vi "Config editor for 19 cluster.vi"() -> ()   [LabVIEW 2022 SP3]
uses:
  085b3232-e767-4131-a9f9-8eb3103b6023.vi
  <vilib>/Utility/file.llb/Read Delimited Spreadsheet (string).vi
  <vilib>/Utility/file.llb/Write Delimited Spreadsheet (string).vi
panel:
  out "AI config 2":T1(array[cluster])=[{"Channel_Name"="G_PT_Press_1", "Channel_Number"="PXI2Slot5/ai1", "Pre_Scale_min"=0.0, "Pre_Scale_max"=10.0, "Sensor_min"=0.0, "Sensor_max"=100.0, "Units"="barg", "VI Category"="AI_V_1KHZ"}, {"Channel_Name"="G_PT_Press_2", "Channel_Number"="PXI2Slot4/ai6", "Pre_Scale_min"=0.004, "Pre_Scale_max"=0.02, "Sensor_min"=0.0, "Sensor_max"=100.0, "Units"="barg", "VI Category"="AI_C_NRT"}, {"Channel_Name"="I_PT(P)_1", "Channel_Number"="PXI2Slot2/ai0", "Pre_Scale_min"=0.004, "Pre_Scale_max"=0.02, "Sensor_min"=0.0, "Sensor_max"=100.0, "Units"="barg", "VI Category"="AI_C_RT"}, {"Channel_Name"="I_PT(P)_2", "Channel_Number"="PXI2Slot2/ai1", "Pre_Scale_min"=0.004, "Pre_Scale_max"=0.02, "Sensor_min"=0.0, "Sensor_max"=100.0, "Units"="barg", "VI Category"="AI_C_RT"}, {"Channel_Name"="I_PT(P)_3", "Channel_Number"="PXI2Slot2/ai2", "Pre_Scale_min"=0.004, "Pre_Scale_max"=0.02, "Sensor_min"=0.0, "Sensor_max"=100.0, "Units"="barg", "VI Category"="AI_C_RT"}, {"Channel_Name"="I_PT(P)_4", "Channel_Number"="PXI2Slot2/ai3", "Pre_Scale_min"=0.004, "Pre_Scale_max"=0.02, "Sensor_min"=0.0, "Sensor_max"=100.0, "Units"="barg", "VI Category"="AI_C_RT"}, {"Channel_Name"="I_PT(P)_5", "Channel_Number"="PXI2Slot2/ai4", "Pre_Scale_min"=0.004, "Pre_Scale_max"=0.02, "Sensor_min"=0.0, "Sensor_max"=100.0, "Units"="barg", "VI Category"="AI_C_RT"}, {"Channel_Name"="I_PT(P)_6", "Channel_Number"="PXI2Slot2/ai5", "Pre_Scale_min"=0.004, "Pre_Scale_max"=0.02, "Sensor_min"=0.0, "Sensor_max"=100.0, "Units"="barg", "VI Category"="AI_C_RT"}, {"Channel_Name"="I_PT(P)_7", "Channel_Number"="PXI2Slot2/ai6", "Pre_Scale_min"=0.004, "Pre_Scale_max"=0.02, "Sensor_min"=0.0, "Sensor_max"=100.0, "Units"="barg", "VI Category"="AI_C_RT"}, {"Channel_Name"="I_PT(P)_8", "Channel_Number"="PXI2Slot2/ai7", "Pre_Scale_min"=0.004, "Pre_Scale_max"=0.02, "Sensor_min"=0.0, "Sensor_max"=100.0, "Units"="barg", "VI Category"="AI_C_RT"}, {"Channel_Name"="I_PT(P)_9", "Channel_Number"="PXI2Slot2/ai8", "Pre_Scale_min"=0.004, "Pre_Scale_max"=0.02, "Sensor_min"=0.0, "Sensor_max"=100.0, "Units"="barg", "VI Category"="AI_C_RT"}, {"Channel_Name"="I_PT(P)_10", "Channel_Number"="PXI2Slot2/ai9", "Pre_Scale_min"=0.004, "Pre_Scale_max"=0.02, "Sensor_min"=0.0, "Sensor_max"=100.0, "Units"="barg", "VI Category"="AI_C_RT"}, {"Channel_Name"="I_PT(P)_11", "Channel_Number"="PXI2Slot2/ai10", "Pre_Scale_min"=0.004, "Pre_Scale_max"=0.02, "Sensor_min"=0.0, "Sensor_max"=100.0, "Units"="barg", "VI Category"="AI_C_RT"}, {"Channel_Name"="I_PT(P)_12", "Channel_Number"="PXI2Slot2/ai11", "Pre_Scale_min"=0.004, "Pre_Scale_max"=0.02, "Sensor_min"=0.0, "Sensor_max"=100.0, "Units"="barg", "VI Category"="AI_C_RT"}, {"Channel_Name"="I_PT(P)_13", "Channel_Number"="PXI2Slot2/ai12", "Pre_Scale_min"=0.004, "Pre_Scale_max"=0.02, "Sensor_min"=0.0, "Sensor_max"=100.0, "Units"="barg", "VI Category"="AI_C_RT"}, {"Channel_Name"="I_PT(P)_14", "Channel_Number"="PXI2Slot2/ai13", "Pre_Scale_min"=0.004, "Pre_Scale_max"=0.02, "Sensor_min"=0.0, "Sensor_max"=100.0, "Units"="barg", "VI Category"="AI_C_RT"}, {"Channel_Name"="I_PT(P)_15", "Channel_Number"="PXI2Slot2/ai14", "Pre_Scale_min"=0.004, "Pre_Scale_max"=0.02, "Sensor_min"=0.0, "Sensor_max"=100.0, "Units"="barg", "VI Category"="AI_C_RT"}, {"Channel_Name"="I_PT(P)_16", "Channel_Number"="PXI2Slot2/ai15", "Pre_Scale_min"=0.004, "Pre_Scale_max"=0.02, "Sensor_min"=0.0, "Sensor_max"=100.0, "Units"="barg", "VI Category"="AI_C_RT"}, {"Channel_Name"="I_PT(P)_17", "Channel_Number"="PXI2Slot2/ai16", "Pre_Scale_min"=0.004, "Pre_Scale_max"=0.02, "Sensor_min"=0.0, "Sensor_max"=100.0, "Units"="barg", "VI Category"="AI_C_RT"}, {"Channel_Name"="I_PT(P)_18", "Channel_Number"="PXI2Slot2/ai17", "Pre_Scale_min"=0.004, "Pre_Scale_max"=0.02, "Sensor_min"=0.0, "Sensor_max"=100.0, "Units"="barg", "VI Category"="AI_C_RT"}, {"Channel_Name"="I_PT(P)_19", "Channel_Number"="PXI2Slot2/ai18", "Pre_Scale_min"=0.004, "Pre_Scale_max"=0.02, "Sensor_min"=0.0, "Sensor_max"=100.0, "Units"="barg", "VI Category"="AI_C_RT"}, {"Channel_Name"="I_PT(Red)_1", "Channel_Number"="PXI2Slot2/ai19", "Pre_Scale_min"=0.004, "Pre_Scale_max"=0.02, "Sensor_min"=0.0, "Sensor_max"=100.0, "Units"="barg", "VI Category"="AI_C_RT"}, {"Channel_Name"="I_PT(Red)_2", "Channel_Number"="PXI2Slot2/ai20", "Pre_Scale_min"=0.004, "Pre_Scale_max"=0.02, "Sensor_min"=0.0, "Sensor_max"=100.0, "Units"="barg", "VI Category"="AI_C_RT"}, {"Channel_Name"="I_PT(Red)_3", "Channel_Number"="PXI2Slot2/ai21", "Pre_Scale_min"=0.004, "Pre_Scale_max"=0.02, "Sensor_min"=0.0, "Sensor_max"=100.0, "Units"="barg", "VI Category"="AI_C_RT"}, {"Channel_Name"="I_PT(Red)_4", "Channel_Number"="PXI2Slot2/ai22", "Pre_Scale_min"=0.004, "Pre_Scale_max"=0.02, "Sensor_min"=0.0, "Sensor_max"=100.0, "Units"="barg", "VI Category"="AI_C_RT"}, {"Channel_Name"="I_PT(Red)_5", "Channel_Number"="PXI2Slot2/ai23", "Pre_Scale_min"=0.004, "Pre_Scale_max"=0.02, "Sensor_min"=0.0, "Sensor_max"=100.0, "Units"="barg", "VI Category"="AI_C_RT"}, {"Channel_Name"="I_PT(Red)_6", "Channel_Number"="PXI2Slot2/ai24", "Pre_Scale_min"=0.004, "Pre_Scale_max"=0.02, "Sensor_min"=0.0, "Sensor_max"=100.0, "Units"="barg", "VI Category"="AI_C_RT"}, {"Channel_Name"="I_PT(Red)_7", "Channel_Number"="PXI2Slot2/ai25", "Pre_Scale_min"=0.004, "Pre_Scale_max"=0.02, "Sensor_min"=0.0, "Sensor_max"=100.0, "Units"="barg", "VI Category"="AI_C_RT"}, {"Channel_Name"="I_PT(Red)_8", "Channel_Number"="PXI2Slot2/ai26", "Pre_Scale_min"=0.004, "Pre_Scale_max"=0.02, "Sensor_min"=0.0, "Sensor_max"=100.0, "Units"="barg", "VI Category"="AI_C_RT"}, {"Channel_Name"="I_PT(Red)_9", "Channel_Number"="PXI2Slot2/ai27", "Pre_Scale_min"=0.004, "Pre_Scale_max"=0.02, "Sensor_min"=0.0, "Sensor_max"=100.0, "Units"="barg", "VI Category"="AI_C_RT"}, {"Channel_Name"="I_PT(Red)_10", "Channel_Number"="PXI2Slot2/ai28", "Pre_Scale_min"=0.004, "Pre_Scale_max"=0.02, "Sensor_min"=0.0, "Sensor_max"=100.0, "Units"="barg", "VI Category"="AI_C_RT"}, {"Channel_Name"="I_PT(Red)_11", "Channel_Number"="PXI2Slot2/ai29", "Pre_Scale_min"=0.004, "Pre_Scale_max"=0.02, "Sensor_min"=0.0, "Sensor_max"=100.0, "Units"="barg", "VI Category"="AI_C_RT"}, {"Channel_Name"="I_PT(Red)_12", "Channel_Number"="PXI2Slot2/ai30", "Pre_Scale_min"=0.004, "Pre_Scale_max"=0.02, "Sensor_min"=0.0, "Sensor_max"=100.0, "Units"="barg", "VI Category"="AI_C_RT"}, {"Channel_Name"="I_PT(Red)_13", "Channel_Number"="PXI2Slot2/ai31", "Pre_Scale_min"=0.004, "Pre_Scale_max"=0.02, "Sensor_min"=0.0, "Sensor_max"=100.0, "Units"="barg", "VI Category"="AI_C_RT"}, {"Channel_Name"="I_PT(Red)_14", "Channel_Number"="PXI2Slot3/ai0", "Pre_Scale_min"=0.004, "Pre_Scale_max"=0.02, "Sensor_min"=0.0, "Sensor_max"=100.0, "Units"="barg", "VI Category"="AI_C_RT"}, {"Channel_Name"="I_PT(Red)_15", "Channel_Number"="PXI2Slot3/ai1", "Pre_Scale_min"=0.004, "Pre_Scale_max"=0.02, "Sensor_min"=0.0, "Sensor_max"=100.0, "Units"="barg", "VI Category"="AI_C_RT"}, {"Channel_Name"="I_PT(Red)_16", "Channel_Number"="PXI2Slot3/ai2", "Pre_Scale_min"=0.004, "Pre_Scale_max"=0.02, "Sensor_min"=0.0, "Sensor_max"=100.0, "Units"="barg", "VI Category"="AI_C_RT"}, {"Channel_Name"="I_PT(Red)_17", "Channel_Number"="PXI2Slot3/ai3", "Pre_Scale_min"=0.004, "Pre_Scale_max"=0.02, "Sensor_min"=0.0, "Sensor_max"=100.0, "Units"="barg", "VI Category"="AI_C_RT"}, {"Channel_Name"="I_PT(Red)_18", "Channel_Number"="PXI2Slot3/ai4", "Pre_Scale_min"=0.004, "Pre_Scale_max"=0.02, "Sensor_min"=0.0, "Sensor_max"=100.0, "Units"="barg", "VI Category"="AI_C_RT"}, {"Channel_Name"="I_PT(Red)_19", "Channel_Number"="PXI2Slot3/ai5", "Pre_Scale_min"=0.004, "Pre_Scale_max"=0.02, "Sensor_min"=0.0, "Sensor_max"=100.0, "Units"="barg", "VI Category"="AI_C_RT"}]
  in  "AI config":T1(array[cluster])=[{"Channel_Name"="G_PT_Press_1", "Channel_Number"="PXI2Slot5/ai1", "Pre_Scale_min"=0.0, "Pre_Scale_max"=10.0, "Sensor_min"=0.0, "Sensor_max"=100.0, "Units"="barg", "VI Category"="AI_V_1KHZ"}, {"Channel_Name"="G_PT_Press_2", "Channel_Number"="PXI2Slot4/ai6", "Pre_Scale_min"=0.004, "Pre_Scale_max"=0.02, "Sensor_min"=0.0, "Sensor_max"=100.0, "Units"="barg", "VI Category"="AI_C_NRT"}, {"Channel_Name"="I_PT(P)_1", "Channel_Number"="PXI2Slot2/ai0", "Pre_Scale_min"=0.004, "Pre_Scale_max"=0.02, "Sensor_min"=0.0, "Sensor_max"=100.0, "Units"="barg", "VI Category"="AI_C_RT"}, {"Channel_Name"="I_PT(P)_2", "Channel_Number"="PXI2Slot2/ai1", "Pre_Scale_min"=0.004, "Pre_Scale_max"=0.02, "Sensor_min"=0.0, "Sensor_max"=100.0, "Units"="barg", "VI Category"="AI_C_RT"}, {"Channel_Name"="I_PT(P)_3", "Channel_Number"="PXI2Slot2/ai2", "Pre_Scale_min"=0.004, "Pre_Scale_max"=0.02, "Sensor_min"=0.0, "Sensor_max"=100.0, "Units"="barg", "VI Category"="AI_C_RT"}, {"Channel_Name"="I_PT(P)_4", "Channel_Number"="PXI2Slot2/ai3", "Pre_Scale_min"=0.004, "Pre_Scale_max"=0.02, "Sensor_min"=0.0, "Sensor_max"=100.0, "Units"="barg", "VI Category"="AI_C_RT"}, {"Channel_Name"="I_PT(P)_5", "Channel_Number"="PXI2Slot2/ai4", "Pre_Scale_min"=0.004, "Pre_Scale_max"=0.02, "Sensor_min"=0.0, "Sensor_max"=100.0, "Units"="barg", "VI Category"="AI_C_RT"}, {"Channel_Name"="I_PT(P)_6", "Channel_Number"="PXI2Slot2/ai5", "Pre_Scale_min"=0.004, "Pre_Scale_max"=0.02, "Sensor_min"=0.0, "Sensor_max"=100.0, "Units"="barg", "VI Category"="AI_C_RT"}, {"Channel_Name"="I_PT(P)_7", "Channel_Number"="PXI2Slot2/ai6", "Pre_Scale_min"=0.004, "Pre_Scale_max"=0.02, "Sensor_min"=0.0, "Sensor_max"=100.0, "Units"="barg", "VI Category"="AI_C_RT"}, {"Channel_Name"="I_PT(P)_8", "Channel_Number"="PXI2Slot2/ai7", "Pre_Scale_min"=0.004, "Pre_Scale_max"=0.02, "Sensor_min"=0.0, "Sensor_max"=100.0, "Units"="barg", "VI Category"="AI_C_RT"}, {"Channel_Name"="I_PT(P)_9", "Channel_Number"="PXI2Slot2/ai8", "Pre_Scale_min"=0.004, "Pre_Scale_max"=0.02, "Sensor_min"=0.0, "Sensor_max"=100.0, "Units"="barg", "VI Category"="AI_C_RT"}, {"Channel_Name"="I_PT(P)_10", "Channel_Number"="PXI2Slot2/ai9", "Pre_Scale_min"=0.004, "Pre_Scale_max"=0.02, "Sensor_min"=0.0, "Sensor_max"=100.0, "Units"="barg", "VI Category"="AI_C_RT"}, {"Channel_Name"="I_PT(P)_11", "Channel_Number"="PXI2Slot2/ai10", "Pre_Scale_min"=0.004, "Pre_Scale_max"=0.02, "Sensor_min"=0.0, "Sensor_max"=100.0, "Units"="barg", "VI Category"="AI_C_RT"}, {"Channel_Name"="I_PT(P)_12", "Channel_Number"="PXI2Slot2/ai11", "Pre_Scale_min"=0.004, "Pre_Scale_max"=0.02, "Sensor_min"=0.0, "Sensor_max"=100.0, "Units"="barg", "VI Category"="AI_C_RT"}, {"Channel_Name"="I_PT(P)_13", "Channel_Number"="PXI2Slot2/ai12", "Pre_Scale_min"=0.004, "Pre_Scale_max"=0.02, "Sensor_min"=0.0, "Sensor_max"=100.0, "Units"="barg", "VI Category"="AI_C_RT"}, {"Channel_Name"="I_PT(P)_14", "Channel_Number"="PXI2Slot2/ai13", "Pre_Scale_min"=0.004, "Pre_Scale_max"=0.02, "Sensor_min"=0.0, "Sensor_max"=100.0, "Units"="barg", "VI Category"="AI_C_RT"}, {"Channel_Name"="I_PT(P)_15", "Channel_Number"="PXI2Slot2/ai14", "Pre_Scale_min"=0.004, "Pre_Scale_max"=0.02, "Sensor_min"=0.0, "Sensor_max"=100.0, "Units"="barg", "VI Category"="AI_C_RT"}, {"Channel_Name"="I_PT(P)_16", "Channel_Number"="PXI2Slot2/ai15", "Pre_Scale_min"=0.004, "Pre_Scale_max"=0.02, "Sensor_min"=0.0, "Sensor_max"=100.0, "Units"="barg", "VI Category"="AI_C_RT"}, {"Channel_Name"="I_PT(P)_17", "Channel_Number"="PXI2Slot2/ai16", "Pre_Scale_min"=0.004, "Pre_Scale_max"=0.02, "Sensor_min"=0.0, "Sensor_max"=100.0, "Units"="barg", "VI Category"="AI_C_RT"}, {"Channel_Name"="I_PT(P)_18", "Channel_Number"="PXI2Slot2/ai17", "Pre_Scale_min"=0.004, "Pre_Scale_max"=0.02, "Sensor_min"=0.0, "Sensor_max"=100.0, "Units"="barg", "VI Category"="AI_C_RT"}, {"Channel_Name"="I_PT(P)_19", "Channel_Number"="PXI2Slot2/ai18", "Pre_Scale_min"=0.004, "Pre_Scale_max"=0.02, "Sensor_min"=0.0, "Sensor_max"=100.0, "Units"="barg", "VI Category"="AI_C_RT"}, {"Channel_Name"="I_PT(Red)_1", "Channel_Number"="PXI2Slot2/ai19", "Pre_Scale_min"=0.004, "Pre_Scale_max"=0.02, "Sensor_min"=0.0, "Sensor_max"=100.0, "Units"="barg", "VI Category"="AI_C_RT"}, {"Channel_Name"="I_PT(Red)_2", "Channel_Number"="PXI2Slot2/ai20", "Pre_Scale_min"=0.004, "Pre_Scale_max"=0.02, "Sensor_min"=0.0, "Sensor_max"=100.0, "Units"="barg", "VI Category"="AI_C_RT"}, {"Channel_Name"="I_PT(Red)_3", "Channel_Number"="PXI2Slot2/ai21", "Pre_Scale_min"=0.004, "Pre_Scale_max"=0.02, "Sensor_min"=0.0, "Sensor_max"=100.0, "Units"="barg", "VI Category"="AI_C_RT"}, {"Channel_Name"="I_PT(Red)_4", "Channel_Number"="PXI2Slot2/ai22", "Pre_Scale_min"=0.004, "Pre_Scale_max"=0.02, "Sensor_min"=0.0, "Sensor_max"=100.0, "Units"="barg", "VI Category"="AI_C_RT"}, {"Channel_Name"="I_PT(Red)_5", "Channel_Number"="PXI2Slot2/ai23", "Pre_Scale_min"=0.004, "Pre_Scale_max"=0.02, "Sensor_min"=0.0, "Sensor_max"=100.0, "Units"="barg", "VI Category"="AI_C_RT"}, {"Channel_Name"="I_PT(Red)_6", "Channel_Number"="PXI2Slot2/ai24", "Pre_Scale_min"=0.004, "Pre_Scale_max"=0.02, "Sensor_min"=0.0, "Sensor_max"=100.0, "Units"="barg", "VI Category"="AI_C_RT"}, {"Channel_Name"="I_PT(Red)_7", "Channel_Number"="PXI2Slot2/ai25", "Pre_Scale_min"=0.004, "Pre_Scale_max"=0.02, "Sensor_min"=0.0, "Sensor_max"=100.0, "Units"="barg", "VI Category"="AI_C_RT"}, {"Channel_Name"="I_PT(Red)_8", "Channel_Number"="PXI2Slot2/ai26", "Pre_Scale_min"=0.004, "Pre_Scale_max"=0.02, "Sensor_min"=0.0, "Sensor_max"=100.0, "Units"="barg", "VI Category"="AI_C_RT"}, {"Channel_Name"="I_PT(Red)_9", "Channel_Number"="PXI2Slot2/ai27", "Pre_Scale_min"=0.004, "Pre_Scale_max"=0.02, "Sensor_min"=0.0, "Sensor_max"=100.0, "Units"="barg", "VI Category"="AI_C_RT"}, {"Channel_Name"="I_PT(Red)_10", "Channel_Number"="PXI2Slot2/ai28", "Pre_Scale_min"=0.004, "Pre_Scale_max"=0.02, "Sensor_min"=0.0, "Sensor_max"=100.0, "Units"="barg", "VI Category"="AI_C_RT"}, {"Channel_Name"="I_PT(Red)_11", "Channel_Number"="PXI2Slot2/ai29", "Pre_Scale_min"=0.004, "Pre_Scale_max"=0.02, "Sensor_min"=0.0, "Sensor_max"=100.0, "Units"="barg", "VI Category"="AI_C_RT"}, {"Channel_Name"="I_PT(Red)_12", "Channel_Number"="PXI2Slot2/ai30", "Pre_Scale_min"=0.004, "Pre_Scale_max"=0.02, "Sensor_min"=0.0, "Sensor_max"=100.0, "Units"="barg", "VI Category"="AI_C_RT"}, {"Channel_Name"="I_PT(Red)_13", "Channel_Number"="PXI2Slot2/ai31", "Pre_Scale_min"=0.004, "Pre_Scale_max"=0.02, "Sensor_min"=0.0, "Sensor_max"=100.0, "Units"="barg", "VI Category"="AI_C_RT"}, {"Channel_Name"="I_PT(Red)_14", "Channel_Number"="PXI2Slot3/ai0", "Pre_Scale_min"=0.004, "Pre_Scale_max"=0.02, "Sensor_min"=0.0, "Sensor_max"=100.0, "Units"="barg", "VI Category"="AI_C_RT"}, {"Channel_Name"="I_PT(Red)_15", "Channel_Number"="PXI2Slot3/ai1", "Pre_Scale_min"=0.004, "Pre_Scale_max"=0.02, "Sensor_min"=0.0, "Sensor_max"=100.0, "Units"="barg", "VI Category"="AI_C_RT"}, {"Channel_Name"="I_PT(Red)_16", "Channel_Number"="PXI2Slot3/ai2", "Pre_Scale_min"=0.004, "Pre_Scale_max"=0.02, "Sensor_min"=0.0, "Sensor_max"=100.0, "Units"="barg", "VI Category"="AI_C_RT"}, {"Channel_Name"="I_PT(Red)_17", "Channel_Number"="PXI2Slot3/ai3", "Pre_Scale_min"=0.004, "Pre_Scale_max"=0.02, "Sensor_min"=0.0, "Sensor_max"=100.0, "Units"="barg", "VI Category"="AI_C_RT"}, {"Channel_Name"="I_PT(Red)_18", "Channel_Number"="PXI2Slot3/ai4", "Pre_Scale_min"=0.004, "Pre_Scale_max"=0.02, "Sensor_min"=0.0, "Sensor_max"=100.0, "Units"="barg", "VI Category"="AI_C_RT"}, {"Channel_Name"="I_PT(Red)_19", "Channel_Number"="PXI2Slot3/ai5", "Pre_Scale_min"=0.004, "Pre_Scale_max"=0.02, "Sensor_min"=0.0, "Sensor_max"=100.0, "Units"="barg", "VI Category"="AI_C_RT"}]
  out "Array 4":string[](array[string])
  out "Strings [] 2":string[](array[string])
  in  "Channel_Name":string(combo)="G_PT_Press_1"
  out "output array":string[][](array[string])
  out "all rows":string[][](array[string])
  in  "file path (dialog if empty)":path
  out "Array 2":string[](array[string])
  out "sorted array":string[](array[string])
  out "DO config 2":T2(array[cluster])
  out "Array":T2(array[cluster])
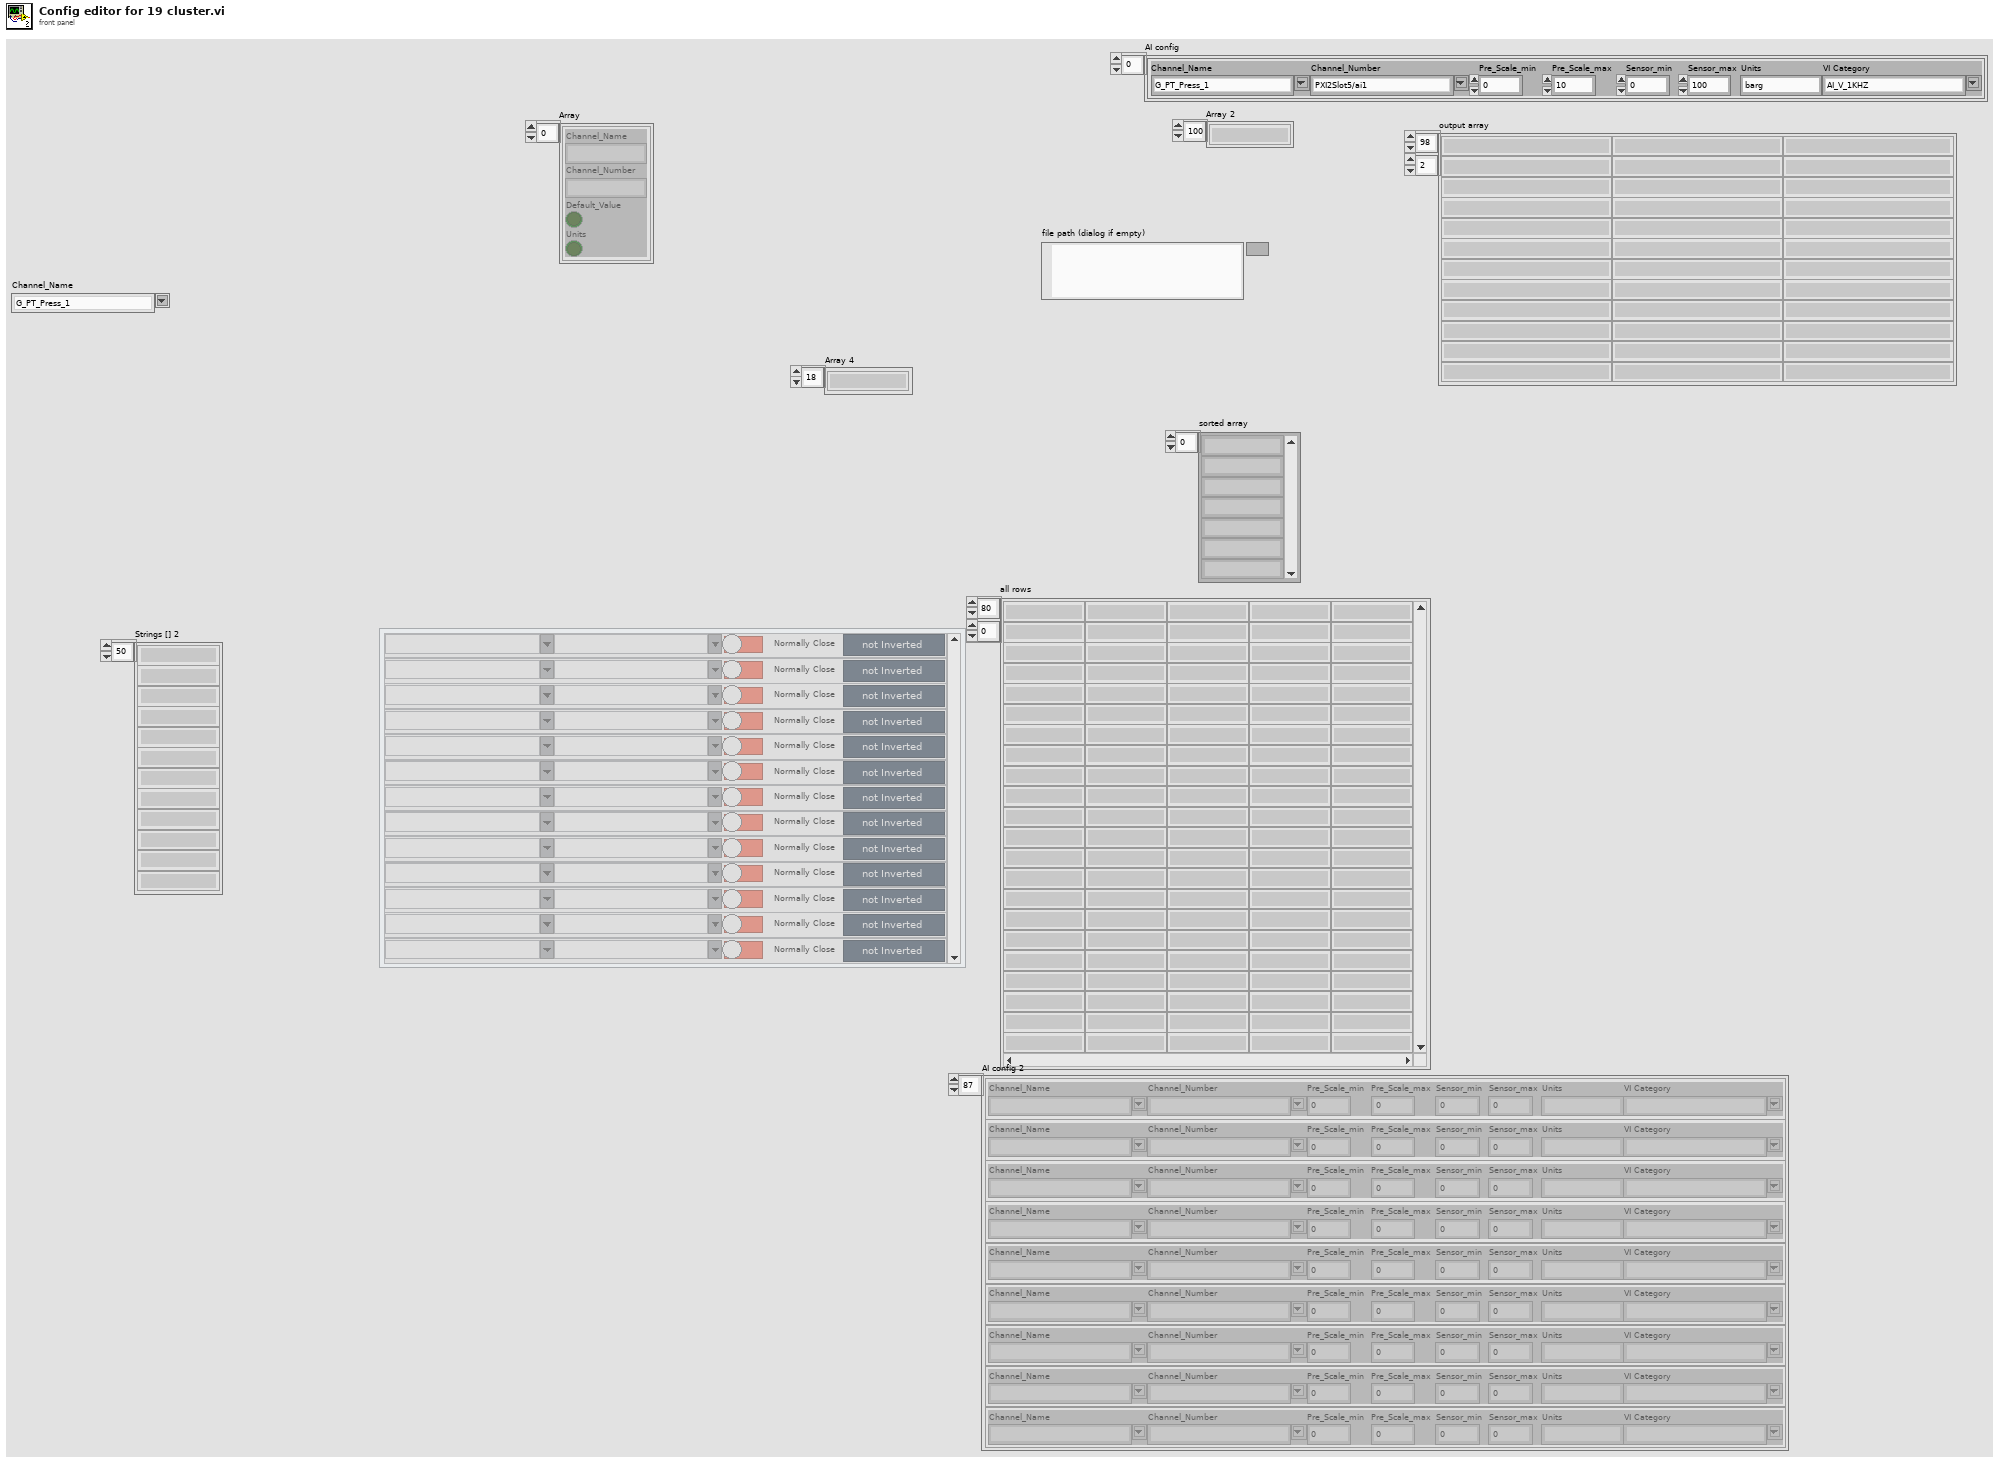
[diagram p1: front panel]
types:
  T1 = cluster{"Channel_Name":string, "Channel_Number":string, "Pre_Scale_min":dbl, "Pre_Scale_max":dbl, "Sensor_min":dbl, "Sensor_max":dbl, "Units":string, "VI Category":string}[]
  T2 = cluster{"Channel_Name":string, "Channel_Number":string, "Default_Value":bool, "Units":bool}[]
  T3 = cluster{"Channel_Name":string, "Channel_Number":string, "Pre_Scale_min":dbl, "Pre_Scale_max":dbl, "Sensor_min":dbl, "Sensor_max":dbl, "Units":string, "VI Category":string}
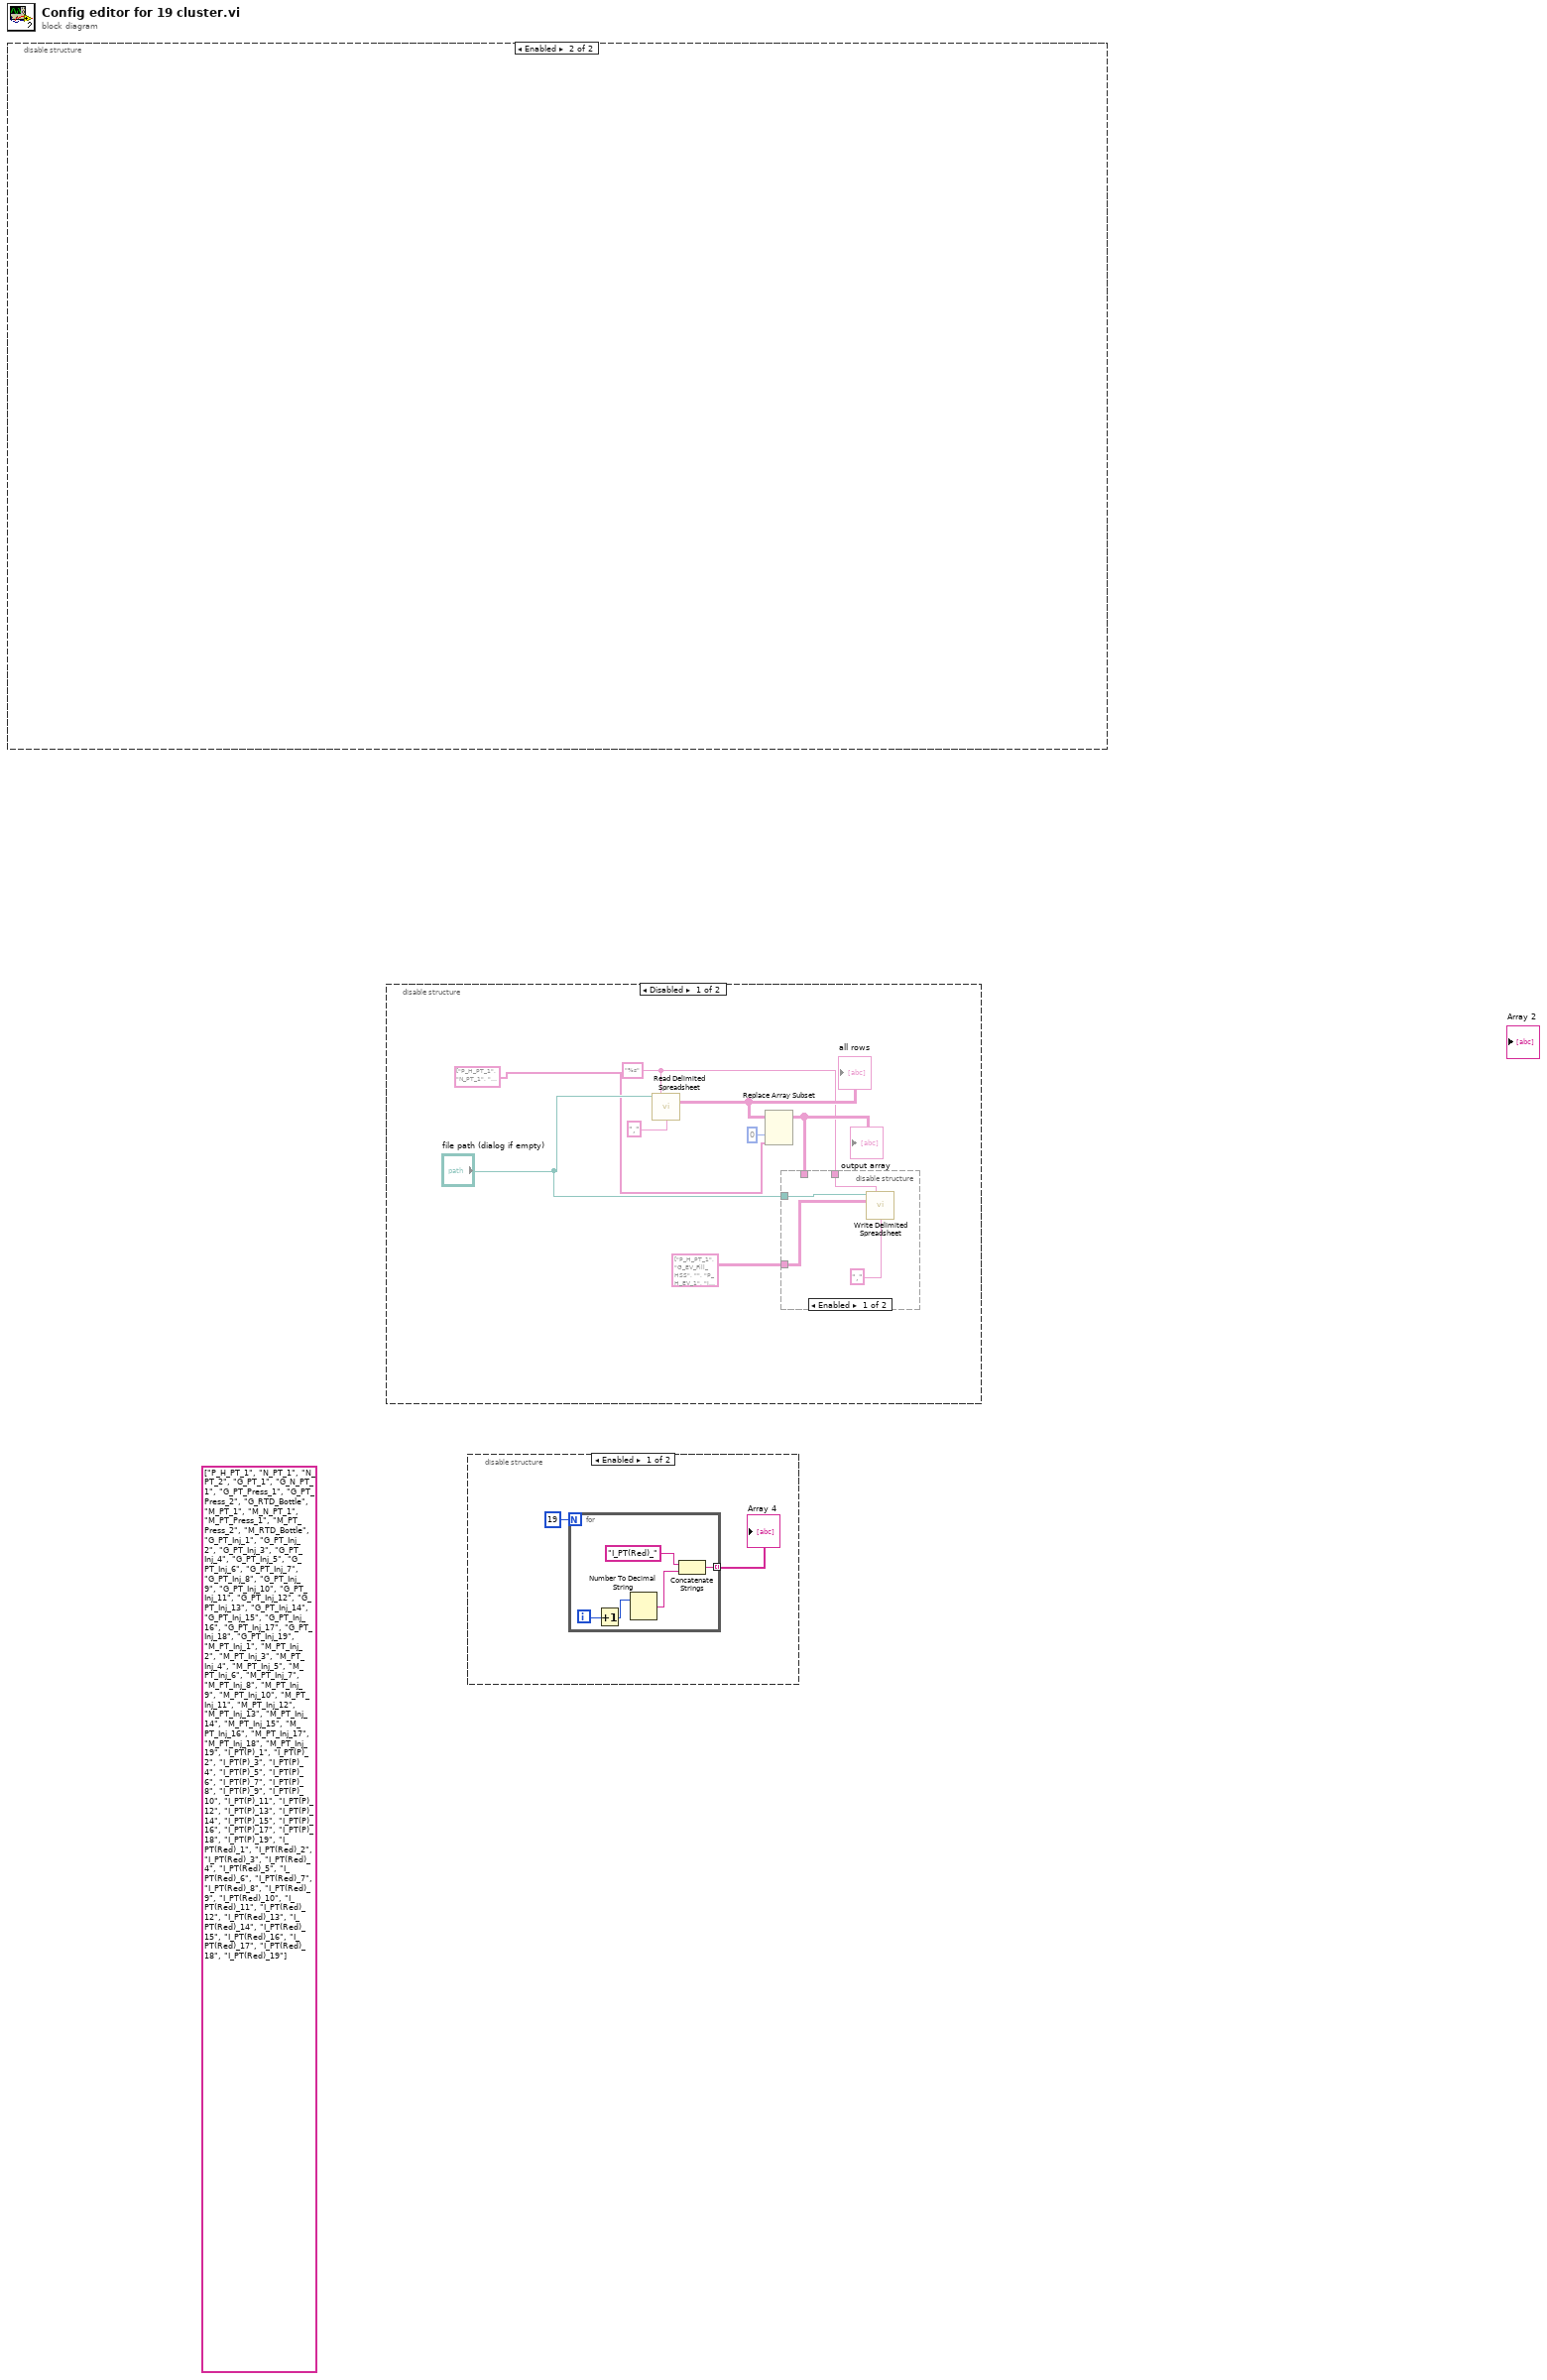
[diagram p0: block diagram]
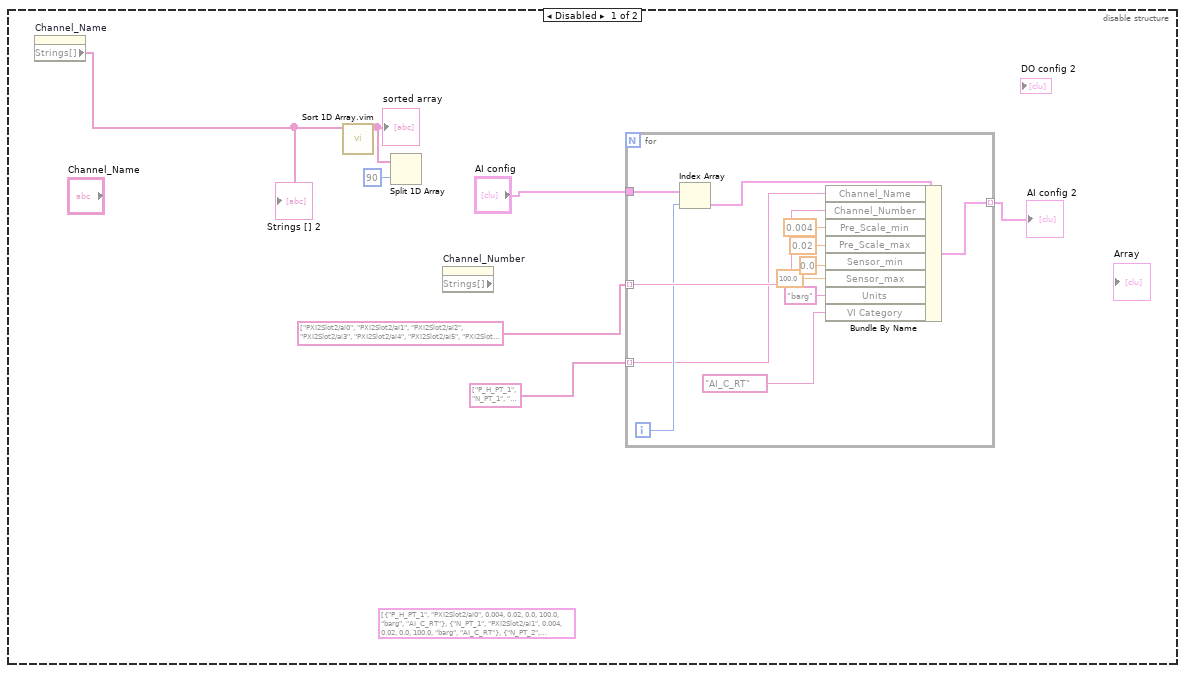
[diagram p3: hidden frame]
diagram:
  (unwired) string[] ["P_H_PT_1", "N_PT_1", "N_PT_2", "G_PT_1", "G_N_PT_1", "G_PT_Press_1", "G_PT_Press_2", "G_RTD_Bottle", "M_PT_1", "M_N_PT_1", "M_PT_Press_1", "M_PT_Press_2", "M_RTD_Bottle", "G_PT_Inj_1", "G_PT_Inj_2", "G_PT_Inj_3", "G_PT_Inj_4", "G_PT_Inj_5", "G_PT_Inj_6", "G_PT_Inj_7", "G_PT_Inj_8", "G_PT_Inj_9", "G_PT_Inj_10", "G_PT_Inj_11", "G_PT_Inj_12", "G_PT_Inj_13", "G_PT_Inj_14", "G_PT_Inj_15", "G_PT_Inj_16", "G_PT_Inj_17", "G_PT_Inj_18", "G_PT_Inj_19", "M_PT_Inj_1", "M_PT_Inj_2", "M_PT_Inj_3", "M_PT_Inj_4", "M_PT_Inj_5", "M_PT_Inj_6", "M_PT_Inj_7", "M_PT_Inj_8", "M_PT_Inj_9", "M_PT_Inj_10", "M_PT_Inj_11", "M_PT_Inj_12", "M_PT_Inj_13", "M_PT_Inj_14", "M_PT_Inj_15", "M_PT_Inj_16", "M_PT_Inj_17", "M_PT_Inj_18", "M_PT_Inj_19", "I_PT(P)_1", "I_PT(P)_2", "I_PT(P)_3", "I_PT(P)_4", "I_PT(P)_5", "I_PT(P)_6", "I_PT(P)_7", "I_PT(P)_8", "I_PT(P)_9", "I_PT(P)_10", "I_PT(P)_11", "I_PT(P)_12", "I_PT(P)_13", "I_PT(P)_14", "I_PT(P)_15", "I_PT(P)_16", "I_PT(P)_17", "I_PT(P)_18", "I_PT(P)_19", "I_PT(Red)_1", "I_PT(Red)_2", "I_PT(Red)_3", "I_PT(Red)_4", "I_PT(Red)_5", "I_PT(Red)_6", "I_PT(Red)_7", "I_PT(Red)_8", "I_PT(Red)_9", "I_PT(Red)_10", "I_PT(Red)_11", "I_PT(Red)_12", "I_PT(Red)_13", "I_PT(Red)_14", "I_PT(Red)_15", "I_PT(Red)_16", "I_PT(Red)_17", "I_PT(Red)_18", "I_PT(Red)_19"] ("appended array 2")
  n1 = disable-structure shown="Enabled" {
    frame Disabled {
      (unwired) T1 [{"Channel_Name"="P_H_PT_1", "Channel_Number"="PXI2Slot2/ai0", "Pre_Scale_min"=0.004, "Pre_Scale_max"=0.02, "Sensor_min"=0.0, "Sensor_max"=100.0, "Units"="barg", "VI Category"="AI_C_RT"}, {"Channel_Name"="N_PT_1", "Channel_Number"="PXI2Slot2/ai1", "Pre_Scale_min"=0.004, "Pre_Scale_max"=0.02, "Sensor_min"=0.0, "Sensor_max"=100.0, "Units"="barg", "VI Category"="AI_C_RT"}, {"Channel_Name"="N_PT_2", "Channel_Number"="PXI2Slot2/ai2", "Pre_Scale_min"=0.004, "Pre_Scale_max"=0.02, "Sensor_min"=0.0, "Sensor_max"=100.0, "Units"="barg", "VI Category"="AI_C_RT"}, {"Channel_Name"="G_PT_1", "Channel_Number"="PXI2Slot2/ai3", "Pre_Scale_min"=0.004, "Pre_Scale_max"=0.02, "Sensor_min"=0.0, "Sensor_max"=100.0, "Units"="barg", "VI Category"="AI_C_RT"}, {"Channel_Name"="G_N_PT_1", "Channel_Number"="PXI2Slot2/ai4", "Pre_Scale_min"=0.004, "Pre_Scale_max"=0.02, "Sensor_min"=0.0, "Sensor_max"=100.0, "Units"="barg", "VI Category"="AI_C_RT"}, {"Channel_Name"="G_PT_Press_1", "Channel_Number"="PXI2Slot2/ai5", "Pre_Scale_min"=0.004, "Pre_Scale_max"=0.02, "Sensor_min"=0.0, "Sensor_max"=100.0, "Units"="barg", "VI Category"="AI_C_RT"}, {"Channel_Name"="G_PT_Press_2", "Channel_Number"="PXI2Slot2/ai6", "Pre_Scale_min"=0.004, "Pre_Scale_max"=0.02, "Sensor_min"=0.0, "Sensor_max"=100.0, "Units"="barg", "VI Category"="AI_C_RT"}, {"Channel_Name"="G_RTD_Bottle", "Channel_Number"="PXI2Slot2/ai7", "Pre_Scale_min"=0.004, "Pre_Scale_max"=0.02, "Sensor_min"=0.0, "Sensor_max"=100.0, "Units"="barg", "VI Category"="AI_C_RT"}, {"Channel_Name"="M_PT_1", "Channel_Number"="PXI2Slot2/ai8", "Pre_Scale_min"=0.004, "Pre_Scale_max"=0.02, "Sensor_min"=0.0, "Sensor_max"=100.0, "Units"="barg", "VI Category"="AI_C_RT"}, {"Channel_Name"="M_N_PT_1", "Channel_Number"="PXI2Slot2/ai9", "Pre_Scale_min"=0.004, "Pre_Scale_max"=0.02, "Sensor_min"=0.0, "Sensor_max"=100.0, "Units"="barg", "VI Category"="AI_C_RT"}, {"Channel_Name"="M_PT_Press_1", "Channel_Number"="PXI2Slot2/ai10", "Pre_Scale_min"=0.004, "Pre_Scale_max"=0.02, "Sensor_min"=0.0, "Sensor_max"=100.0, "Units"="barg", "VI Category"="AI_C_RT"}, {"Channel_Name"="M_PT_Press_2", "Channel_Number"="PXI2Slot2/ai11", "Pre_Scale_min"=0.004, "Pre_Scale_max"=0.02, "Sensor_min"=0.0, "Sensor_max"=100.0, "Units"="barg", "VI Category"="AI_C_RT"}, {"Channel_Name"="M_RTD_Bottle", "Channel_Number"="PXI2Slot2/ai12", "Pre_Scale_min"=0.004, "Pre_Scale_max"=0.02, "Sensor_min"=0.0, "Sensor_max"=100.0, "Units"="barg", "VI Category"="AI_C_RT"}, {"Channel_Name"="G_PT_Inj_1", "Channel_Number"="PXI2Slot2/ai13", "Pre_Scale_min"=0.004, "Pre_Scale_max"=0.02, "Sensor_min"=0.0, "Sensor_max"=100.0, "Units"="barg", "VI Category"="AI_C_RT"}, {"Channel_Name"="G_PT_Inj_2", "Channel_Number"="PXI2Slot2/ai14", "Pre_Scale_min"=0.004, "Pre_Scale_max"=0.02, "Sensor_min"=0.0, "Sensor_max"=100.0, "Units"="barg", "VI Category"="AI_C_RT"}, {"Channel_Name"="G_PT_Inj_3", "Channel_Number"="PXI2Slot2/ai15", "Pre_Scale_min"=0.004, "Pre_Scale_max"=0.02, "Sensor_min"=0.0, "Sensor_max"=100.0, "Units"="barg", "VI Category"="AI_C_RT"}, {"Channel_Name"="G_PT_Inj_4", "Channel_Number"="PXI2Slot2/ai16", "Pre_Scale_min"=0.004, "Pre_Scale_max"=0.02, "Sensor_min"=0.0, "Sensor_max"=100.0, "Units"="barg", "VI Category"="AI_C_RT"}, {"Channel_Name"="G_PT_Inj_5", "Channel_Number"="PXI2Slot2/ai17", "Pre_Scale_min"=0.004, "Pre_Scale_max"=0.02, "Sensor_min"=0.0, "Sensor_max"=100.0, "Units"="barg", "VI Category"="AI_C_RT"}, {"Channel_Name"="G_PT_Inj_6", "Channel_Number"="PXI2Slot2/ai18", "Pre_Scale_min"=0.004, "Pre_Scale_max"=0.02, "Sensor_min"=0.0, "Sensor_max"=100.0, "Units"="barg", "VI Category"="AI_C_RT"}, {"Channel_Name"="G_PT_Inj_7", "Channel_Number"="PXI2Slot2/ai19", "Pre_Scale_min"=0.004, "Pre_Scale_max"=0.02, "Sensor_min"=0.0, "Sensor_max"=100.0, "Units"="barg", "VI Category"="AI_C_RT"}, {"Channel_Name"="G_PT_Inj_8", "Channel_Number"="PXI2Slot2/ai20", "Pre_Scale_min"=0.004, "Pre_Scale_max"=0.02, "Sensor_min"=0.0, "Sensor_max"=100.0, "Units"="barg", "VI Category"="AI_C_RT"}, {"Channel_Name"="G_PT_Inj_9", "Channel_Number"="PXI2Slot2/ai21", "Pre_Scale_min"=0.004, "Pre_Scale_max"=0.02, "Sensor_min"=0.0, "Sensor_max"=100.0, "Units"="barg", "VI Category"="AI_C_RT"}, {"Channel_Name"="G_PT_Inj_10", "Channel_Number"="PXI2Slot2/ai22", "Pre_Scale_min"=0.004, "Pre_Scale_max"=0.02, "Sensor_min"=0.0, "Sensor_max"=100.0, "Units"="barg", "VI Category"="AI_C_RT"}, {"Channel_Name"="G_PT_Inj_11", "Channel_Number"="PXI2Slot2/ai23", "Pre_Scale_min"=0.004, "Pre_Scale_max"=0.02, "Sensor_min"=0.0, "Sensor_max"=100.0, "Units"="barg", "VI Category"="AI_C_RT"}, {"Channel_Name"="G_PT_Inj_12", "Channel_Number"="PXI2Slot2/ai24", "Pre_Scale_min"=0.004, "Pre_Scale_max"=0.02, "Sensor_min"=0.0, "Sensor_max"=100.0, "Units"="barg", "VI Category"="AI_C_RT"}, {"Channel_Name"="G_PT_Inj_13", "Channel_Number"="PXI2Slot2/ai25", "Pre_Scale_min"=0.004, "Pre_Scale_max"=0.02, "Sensor_min"=0.0, "Sensor_max"=100.0, "Units"="barg", "VI Category"="AI_C_RT"}, {"Channel_Name"="G_PT_Inj_14", "Channel_Number"="PXI2Slot2/ai26", "Pre_Scale_min"=0.004, "Pre_Scale_max"=0.02, "Sensor_min"=0.0, "Sensor_max"=100.0, "Units"="barg", "VI Category"="AI_C_RT"}, {"Channel_Name"="G_PT_Inj_15", "Channel_Number"="PXI2Slot2/ai27", "Pre_Scale_min"=0.004, "Pre_Scale_max"=0.02, "Sensor_min"=0.0, "Sensor_max"=100.0, "Units"="barg", "VI Category"="AI_C_RT"}, {"Channel_Name"="G_PT_Inj_16", "Channel_Number"="PXI2Slot2/ai28", "Pre_Scale_min"=0.004, "Pre_Scale_max"=0.02, "Sensor_min"=0.0, "Sensor_max"=100.0, "Units"="barg", "VI Category"="AI_C_RT"}, {"Channel_Name"="G_PT_Inj_17", "Channel_Number"="PXI2Slot2/ai29", "Pre_Scale_min"=0.004, "Pre_Scale_max"=0.02, "Sensor_min"=0.0, "Sensor_max"=100.0, "Units"="barg", "VI Category"="AI_C_RT"}, {"Channel_Name"="G_PT_Inj_18", "Channel_Number"="PXI2Slot2/ai30", "Pre_Scale_min"=0.004, "Pre_Scale_max"=0.02, "Sensor_min"=0.0, "Sensor_max"=100.0, "Units"="barg", "VI Category"="AI_C_RT"}, {"Channel_Name"="G_PT_Inj_19", "Channel_Number"="PXI2Slot2/ai31", "Pre_Scale_min"=0.004, "Pre_Scale_max"=0.02, "Sensor_min"=0.0, "Sensor_max"=100.0, "Units"="barg", "VI Category"="AI_C_RT"}, {"Channel_Name"="M_PT_Inj_1", "Channel_Number"="PXI2Slot3/ai0", "Pre_Scale_min"=0.004, "Pre_Scale_max"=0.02, "Sensor_min"=0.0, "Sensor_max"=100.0, "Units"="barg", "VI Category"="AI_C_RT"}, {"Channel_Name"="M_PT_Inj_2", "Channel_Number"="PXI2Slot3/ai1", "Pre_Scale_min"=0.004, "Pre_Scale_max"=0.02, "Sensor_min"=0.0, "Sensor_max"=100.0, "Units"="barg", "VI Category"="AI_C_RT"}, {"Channel_Name"="M_PT_Inj_3", "Channel_Number"="PXI2Slot3/ai2", "Pre_Scale_min"=0.004, "Pre_Scale_max"=0.02, "Sensor_min"=0.0, "Sensor_max"=100.0, "Units"="barg", "VI Category"="AI_C_RT"}, {"Channel_Name"="M_PT_Inj_4", "Channel_Number"="PXI2Slot3/ai3", "Pre_Scale_min"=0.004, "Pre_Scale_max"=0.02, "Sensor_min"=0.0, "Sensor_max"=100.0, "Units"="barg", "VI Category"="AI_C_RT"}, {"Channel_Name"="M_PT_Inj_5", "Channel_Number"="PXI2Slot3/ai4", "Pre_Scale_min"=0.004, "Pre_Scale_max"=0.02, "Sensor_min"=0.0, "Sensor_max"=100.0, "Units"="barg", "VI Category"="AI_C_RT"}, {"Channel_Name"="M_PT_Inj_6", "Channel_Number"="PXI2Slot3/ai5", "Pre_Scale_min"=0.004, "Pre_Scale_max"=0.02, "Sensor_min"=0.0, "Sensor_max"=100.0, "Units"="barg", "VI Category"="AI_C_RT"}, {"Channel_Name"="M_PT_Inj_7", "Channel_Number"="PXI2Slot3/ai6", "Pre_Scale_min"=0.004, "Pre_Scale_max"=0.02, "Sensor_min"=0.0, "Sensor_max"=100.0, "Units"="barg", "VI Category"="AI_C_RT"}, {"Channel_Name"="M_PT_Inj_8", "Channel_Number"="PXI2Slot3/ai7", "Pre_Scale_min"=0.004, "Pre_Scale_max"=0.02, "Sensor_min"=0.0, "Sensor_max"=100.0, "Units"="barg", "VI Category"="AI_C_RT"}, {"Channel_Name"="M_PT_Inj_9", "Channel_Number"="PXI2Slot3/ai8", "Pre_Scale_min"=0.004, "Pre_Scale_max"=0.02, "Sensor_min"=0.0, "Sensor_max"=100.0, "Units"="barg", "VI Category"="AI_C_RT"}, {"Channel_Name"="M_PT_Inj_10", "Channel_Number"="PXI2Slot3/ai9", "Pre_Scale_min"=0.004, "Pre_Scale_max"=0.02, "Sensor_min"=0.0, "Sensor_max"=100.0, "Units"="barg", "VI Category"="AI_C_RT"}, {"Channel_Name"="M_PT_Inj_11", "Channel_Number"="PXI2Slot3/ai10", "Pre_Scale_min"=0.004, "Pre_Scale_max"=0.02, "Sensor_min"=0.0, "Sensor_max"=100.0, "Units"="barg", "VI Category"="AI_C_RT"}, {"Channel_Name"="M_PT_Inj_12", "Channel_Number"="PXI2Slot3/ai11", "Pre_Scale_min"=0.004, "Pre_Scale_max"=0.02, "Sensor_min"=0.0, "Sensor_max"=100.0, "Units"="barg", "VI Category"="AI_C_RT"}, {"Channel_Name"="M_PT_Inj_13", "Channel_Number"="PXI2Slot3/ai12", "Pre_Scale_min"=0.004, "Pre_Scale_max"=0.02, "Sensor_min"=0.0, "Sensor_max"=100.0, "Units"="barg", "VI Category"="AI_C_RT"}, {"Channel_Name"="M_PT_Inj_14", "Channel_Number"="PXI2Slot3/ai13", "Pre_Scale_min"=0.004, "Pre_Scale_max"=0.02, "Sensor_min"=0.0, "Sensor_max"=100.0, "Units"="barg", "VI Category"="AI_C_RT"}, {"Channel_Name"="M_PT_Inj_15", "Channel_Number"="PXI2Slot3/ai14", "Pre_Scale_min"=0.004, "Pre_Scale_max"=0.02, "Sensor_min"=0.0, "Sensor_max"=100.0, "Units"="barg", "VI Category"="AI_C_RT"}, {"Channel_Name"="M_PT_Inj_16", "Channel_Number"="PXI2Slot3/ai15", "Pre_Scale_min"=0.004, "Pre_Scale_max"=0.02, "Sensor_min"=0.0, "Sensor_max"=100.0, "Units"="barg", "VI Category"="AI_C_RT"}, {"Channel_Name"="M_PT_Inj_17", "Channel_Number"="PXI2Slot3/ai16", "Pre_Scale_min"=0.004, "Pre_Scale_max"=0.02, "Sensor_min"=0.0, "Sensor_max"=100.0, "Units"="barg", "VI Category"="AI_C_RT"}, {"Channel_Name"="M_PT_Inj_18", "Channel_Number"="PXI2Slot3/ai17", "Pre_Scale_min"=0.004, "Pre_Scale_max"=0.02, "Sensor_min"=0.0, "Sensor_max"=100.0, "Units"="barg", "VI Category"="AI_C_RT"}, {"Channel_Name"="M_PT_Inj_19", "Channel_Number"="PXI2Slot3/ai18", "Pre_Scale_min"=0.004, "Pre_Scale_max"=0.02, "Sensor_min"=0.0, "Sensor_max"=100.0, "Units"="barg", "VI Category"="AI_C_RT"}, {"Channel_Name"="I_PT(P)_1", "Channel_Number"="PXI2Slot3/ai19", "Pre_Scale_min"=0.004, "Pre_Scale_max"=0.02, "Sensor_min"=0.0, "Sensor_max"=100.0, "Units"="barg", "VI Category"="AI_C_RT"}, {"Channel_Name"="I_PT(P)_2", "Channel_Number"="PXI2Slot3/ai20", "Pre_Scale_min"=0.004, "Pre_Scale_max"=0.02, "Sensor_min"=0.0, "Sensor_max"=100.0, "Units"="barg", "VI Category"="AI_C_RT"}, {"Channel_Name"="I_PT(P)_3", "Channel_Number"="PXI2Slot3/ai21", "Pre_Scale_min"=0.004, "Pre_Scale_max"=0.02, "Sensor_min"=0.0, "Sensor_max"=100.0, "Units"="barg", "VI Category"="AI_C_RT"}, {"Channel_Name"="I_PT(P)_4", "Channel_Number"="PXI2Slot3/ai22", "Pre_Scale_min"=0.004, "Pre_Scale_max"=0.02, "Sensor_min"=0.0, "Sensor_max"=100.0, "Units"="barg", "VI Category"="AI_C_RT"}, {"Channel_Name"="I_PT(P)_5", "Channel_Number"="PXI2Slot3/ai23", "Pre_Scale_min"=0.004, "Pre_Scale_max"=0.02, "Sensor_min"=0.0, "Sensor_max"=100.0, "Units"="barg", "VI Category"="AI_C_RT"}, {"Channel_Name"="I_PT(P)_6", "Channel_Number"="PXI2Slot3/ai24", "Pre_Scale_min"=0.004, "Pre_Scale_max"=0.02, "Sensor_min"=0.0, "Sensor_max"=100.0, "Units"="barg", "VI Category"="AI_C_RT"}, {"Channel_Name"="I_PT(P)_7", "Channel_Number"="PXI2Slot3/ai25", "Pre_Scale_min"=0.004, "Pre_Scale_max"=0.02, "Sensor_min"=0.0, "Sensor_max"=100.0, "Units"="barg", "VI Category"="AI_C_RT"}, {"Channel_Name"="I_PT(P)_8", "Channel_Number"="PXI2Slot3/ai26", "Pre_Scale_min"=0.004, "Pre_Scale_max"=0.02, "Sensor_min"=0.0, "Sensor_max"=100.0, "Units"="barg", "VI Category"="AI_C_RT"}, {"Channel_Name"="I_PT(P)_9", "Channel_Number"="PXI2Slot3/ai27", "Pre_Scale_min"=0.004, "Pre_Scale_max"=0.02, "Sensor_min"=0.0, "Sensor_max"=100.0, "Units"="barg", "VI Category"="AI_C_RT"}, {"Channel_Name"="I_PT(P)_10", "Channel_Number"="PXI2Slot3/ai28", "Pre_Scale_min"=0.004, "Pre_Scale_max"=0.02, "Sensor_min"=0.0, "Sensor_max"=100.0, "Units"="barg", "VI Category"="AI_C_RT"}, {"Channel_Name"="I_PT(P)_11", "Channel_Number"="PXI2Slot3/ai29", "Pre_Scale_min"=0.004, "Pre_Scale_max"=0.02, "Sensor_min"=0.0, "Sensor_max"=100.0, "Units"="barg", "VI Category"="AI_C_RT"}, {"Channel_Name"="I_PT(P)_12", "Channel_Number"="PXI2Slot3/ai30", "Pre_Scale_min"=0.004, "Pre_Scale_max"=0.02, "Sensor_min"=0.0, "Sensor_max"=100.0, "Units"="barg", "VI Category"="AI_C_RT"}, {"Channel_Name"="I_PT(P)_13", "Channel_Number"="PXI2Slot3/ai31", "Pre_Scale_min"=0.004, "Pre_Scale_max"=0.02, "Sensor_min"=0.0, "Sensor_max"=100.0, "Units"="barg", "VI Category"="AI_C_RT"}, {"Channel_Name"="I_PT(P)_14", "Channel_Number"="PXI2Slot4/ai0", "Pre_Scale_min"=0.004, "Pre_Scale_max"=0.02, "Sensor_min"=0.0, "Sensor_max"=100.0, "Units"="barg", "VI Category"="AI_C_RT"}, {"Channel_Name"="I_PT(P)_15", "Channel_Number"="PXI2Slot4/ai1", "Pre_Scale_min"=0.004, "Pre_Scale_max"=0.02, "Sensor_min"=0.0, "Sensor_max"=100.0, "Units"="barg", "VI Category"="AI_C_RT"}, {"Channel_Name"="I_PT(P)_16", "Channel_Number"="PXI2Slot4/ai2", "Pre_Scale_min"=0.004, "Pre_Scale_max"=0.02, "Sensor_min"=0.0, "Sensor_max"=100.0, "Units"="barg", "VI Category"="AI_C_RT"}, {"Channel_Name"="I_PT(P)_17", "Channel_Number"="PXI2Slot4/ai3", "Pre_Scale_min"=0.004, "Pre_Scale_max"=0.02, "Sensor_min"=0.0, "Sensor_max"=100.0, "Units"="barg", "VI Category"="AI_C_RT"}, {"Channel_Name"="I_PT(P)_18", "Channel_Number"="PXI2Slot4/ai4", "Pre_Scale_min"=0.004, "Pre_Scale_max"=0.02, "Sensor_min"=0.0, "Sensor_max"=100.0, "Units"="barg", "VI Category"="AI_C_RT"}, {"Channel_Name"="I_PT(P)_19", "Channel_Number"="PXI2Slot4/ai5", "Pre_Scale_min"=0.004, "Pre_Scale_max"=0.02, "Sensor_min"=0.0, "Sensor_max"=100.0, "Units"="barg", "VI Category"="AI_C_RT"}, {"Channel_Name"="I_PT(Red)_1", "Channel_Number"="PXI2Slot4/ai6", "Pre_Scale_min"=0.004, "Pre_Scale_max"=0.02, "Sensor_min"=0.0, "Sensor_max"=100.0, "Units"="barg", "VI Category"="AI_C_RT"}, {"Channel_Name"="I_PT(Red)_2", "Channel_Number"="PXI2Slot4/ai7", "Pre_Scale_min"=0.004, "Pre_Scale_max"=0.02, "Sensor_min"=0.0, "Sensor_max"=100.0, "Units"="barg", "VI Category"="AI_C_RT"}, {"Channel_Name"="I_PT(Red)_3", "Channel_Number"="PXI2Slot4/ai8", "Pre_Scale_min"=0.004, "Pre_Scale_max"=0.02, "Sensor_min"=0.0, "Sensor_max"=100.0, "Units"="barg", "VI Category"="AI_C_RT"}, {"Channel_Name"="I_PT(Red)_4", "Channel_Number"="PXI2Slot4/ai9", "Pre_Scale_min"=0.004, "Pre_Scale_max"=0.02, "Sensor_min"=0.0, "Sensor_max"=100.0, "Units"="barg", "VI Category"="AI_C_RT"}, {"Channel_Name"="I_PT(Red)_5", "Channel_Number"="PXI2Slot4/ai10", "Pre_Scale_min"=0.004, "Pre_Scale_max"=0.02, "Sensor_min"=0.0, "Sensor_max"=100.0, "Units"="barg", "VI Category"="AI_C_RT"}, {"Channel_Name"="I_PT(Red)_6", "Channel_Number"="PXI2Slot4/ai11", "Pre_Scale_min"=0.004, "Pre_Scale_max"=0.02, "Sensor_min"=0.0, "Sensor_max"=100.0, "Units"="barg", "VI Category"="AI_C_RT"}, {"Channel_Name"="I_PT(Red)_7", "Channel_Number"="PXI2Slot4/ai12", "Pre_Scale_min"=0.004, "Pre_Scale_max"=0.02, "Sensor_min"=0.0, "Sensor_max"=100.0, "Units"="barg", "VI Category"="AI_C_RT"}, {"Channel_Name"="I_PT(Red)_8", "Channel_Number"="PXI2Slot4/ai13", "Pre_Scale_min"=0.004, "Pre_Scale_max"=0.02, "Sensor_min"=0.0, "Sensor_max"=100.0, "Units"="barg", "VI Category"="AI_C_RT"}, {"Channel_Name"="I_PT(Red)_9", "Channel_Number"="PXI2Slot4/ai14", "Pre_Scale_min"=0.004, "Pre_Scale_max"=0.02, "Sensor_min"=0.0, "Sensor_max"=100.0, "Units"="barg", "VI Category"="AI_C_RT"}, {"Channel_Name"="I_PT(Red)_10", "Channel_Number"="PXI2Slot4/ai15", "Pre_Scale_min"=0.004, "Pre_Scale_max"=0.02, "Sensor_min"=0.0, "Sensor_max"=100.0, "Units"="barg", "VI Category"="AI_C_RT"}, {"Channel_Name"="I_PT(Red)_11", "Channel_Number"="PXI2Slot4/ai16", "Pre_Scale_min"=0.004, "Pre_Scale_max"=0.02, "Sensor_min"=0.0, "Sensor_max"=100.0, "Units"="barg", "VI Category"="AI_C_RT"}, {"Channel_Name"="I_PT(Red)_12", "Channel_Number"="PXI2Slot4/ai17", "Pre_Scale_min"=0.004, "Pre_Scale_max"=0.02, "Sensor_min"=0.0, "Sensor_max"=100.0, "Units"="barg", "VI Category"="AI_C_RT"}, {"Channel_Name"="I_PT(Red)_13", "Channel_Number"="PXI2Slot4/ai18", "Pre_Scale_min"=0.004, "Pre_Scale_max"=0.02, "Sensor_min"=0.0, "Sensor_max"=100.0, "Units"="barg", "VI Category"="AI_C_RT"}, {"Channel_Name"="I_PT(Red)_14", "Channel_Number"="PXI2Slot4/ai19", "Pre_Scale_min"=0.004, "Pre_Scale_max"=0.02, "Sensor_min"=0.0, "Sensor_max"=100.0, "Units"="barg", "VI Category"="AI_C_RT"}, {"Channel_Name"="I_PT(Red)_15", "Channel_Number"="PXI2Slot4/ai20", "Pre_Scale_min"=0.004, "Pre_Scale_max"=0.02, "Sensor_min"=0.0, "Sensor_max"=100.0, "Units"="barg", "VI Category"="AI_C_RT"}, {"Channel_Name"="I_PT(Red)_16", "Channel_Number"="PXI2Slot4/ai21", "Pre_Scale_min"=0.004, "Pre_Scale_max"=0.02, "Sensor_min"=0.0, "Sensor_max"=100.0, "Units"="barg", "VI Category"="AI_C_RT"}, {"Channel_Name"="I_PT(Red)_17", "Channel_Number"="PXI2Slot4/ai22", "Pre_Scale_min"=0.004, "Pre_Scale_max"=0.02, "Sensor_min"=0.0, "Sensor_max"=100.0, "Units"="barg", "VI Category"="AI_C_RT"}, {"Channel_Name"="I_PT(Red)_18", "Channel_Number"="PXI2Slot4/ai23", "Pre_Scale_min"=0.004, "Pre_Scale_max"=0.02, "Sensor_min"=0.0, "Sensor_max"=100.0, "Units"="barg", "VI Category"="AI_C_RT"}, {"Channel_Name"="I_PT(Red)_19", "Channel_Number"="PXI2Slot4/ai24", "Pre_Scale_min"=0.004, "Pre_Scale_max"=0.02, "Sensor_min"=0.0, "Sensor_max"=100.0, "Units"="barg", "VI Category"="AI_C_RT"}] ("AI config 2")
      n2 = property on="Channel_Name" class="CmbBox"() -> ("Strings[]"=w5:string[])  [unwired: 2 in, 2 out]
      "Strings [] 2" <- w5
      n3 = call "Sort 1D Array.vim"("unsorted array"=w5) -> ("sorted array"=w7:string[])  [unwired: 10 in]
      "sorted array" <- w7
      n4 = Split 1D Array(array=w7, index=90) -> ()  [unwired: 2 out]
      n5 = property on="Channel_Number" class="CmbBox" props=["Strings[]"]() -> ()  [unwired: 2 in, 3 out]
      n6 = for {
        tunnel: string[] ["PXI2Slot2/ai0", "PXI2Slot2/ai1", "PXI2Slot2/ai2", "PXI2Slot2/ai3", "PXI2Slot2/ai4", "PXI2Slot2/ai5", "PXI2Slot2/ai6", "PXI2Slot2/ai7", "PXI2Slot2/ai8", "PXI2Slot2/ai9", "PXI2Slot2/ai10", "PXI2Slot2/ai11", "PXI2Slot2/ai12", "PXI2Slot2/ai13", "PXI2Slot2/ai14", "PXI2Slot2/ai15", "PXI2Slot2/ai16", "PXI2Slot2/ai17", "PXI2Slot2/ai18", "PXI2Slot2/ai19", "PXI2Slot2/ai20", "PXI2Slot2/ai21", "PXI2Slot2/ai22", "PXI2Slot2/ai23", "PXI2Slot2/ai24", "PXI2Slot2/ai25", "PXI2Slot2/ai26", "PXI2Slot2/ai27", "PXI2Slot2/ai28", "PXI2Slot2/ai29", "PXI2Slot2/ai30", "PXI2Slot2/ai31", "PXI2Slot3/ai0", "PXI2Slot3/ai1", "PXI2Slot3/ai2", "PXI2Slot3/ai3", "PXI2Slot3/ai4", "PXI2Slot3/ai5", "PXI2Slot3/ai6", "PXI2Slot3/ai7", "PXI2Slot3/ai8", "PXI2Slot3/ai9", "PXI2Slot3/ai10", "PXI2Slot3/ai11", "PXI2Slot3/ai12", "PXI2Slot3/ai13", "PXI2Slot3/ai14", "PXI2Slot3/ai15", "PXI2Slot3/ai16", "PXI2Slot3/ai17", "PXI2Slot3/ai18", "PXI2Slot3/ai19", "PXI2Slot3/ai20", "PXI2Slot3/ai21", "PXI2Slot3/ai22", "PXI2Slot3/ai23", "PXI2Slot3/ai24", "PXI2Slot3/ai25", "PXI2Slot3/ai26", "PXI2Slot3/ai27", "PXI2Slot3/ai28", "PXI2Slot3/ai29", "PXI2Slot3/ai30", "PXI2Slot3/ai31", "PXI2Slot4/ai0", "PXI2Slot4/ai1", "PXI2Slot4/ai2", "PXI2Slot4/ai3", "PXI2Slot4/ai4", "PXI2Slot4/ai5", "PXI2Slot4/ai6", "PXI2Slot4/ai7", "PXI2Slot4/ai8", "PXI2Slot4/ai9", "PXI2Slot4/ai10", "PXI2Slot4/ai11", "PXI2Slot4/ai12", "PXI2Slot4/ai13", "PXI2Slot4/ai14", "PXI2Slot4/ai15", "PXI2Slot4/ai16", "PXI2Slot4/ai17", "PXI2Slot4/ai18", "PXI2Slot4/ai19", "PXI2Slot4/ai20", "PXI2Slot4/ai21", "PXI2Slot4/ai22", "PXI2Slot4/ai23", "PXI2Slot4/ai24", "PXI2Slot4/ai25", "PXI2Slot4/ai26", "PXI2Slot4/ai27", "PXI2Slot4/ai28", "PXI2Slot4/ai29", "PXI2Slot4/ai30", "PXI2Slot4/ai31", "PXI2Slot5/ai0", "PXI2Slot5/ai1", "PXI2Slot5/ai2", "PXI2Slot5/ai3", "PXI2Slot5/ai4", "PXI2Slot5/ai5", "PXI2Slot5/ai6", "PXI2Slot5/ai7", "PXI2Slot5/ai8", "PXI2Slot5/ai9", "PXI2Slot5/ai10", "PXI2Slot5/ai11", "PXI2Slot5/ai12", "PXI2Slot5/ai13", "PXI2Slot5/ai14", "PXI2Slot5/ai15", "PXI2Slot5/ai16", "PXI2Slot5/ai17", "PXI2Slot5/ai18", "PXI2Slot5/ai19", "PXI2Slot5/ai20", "PXI2Slot5/ai21", "PXI2Slot5/ai22", "PXI2Slot5/ai23", "PXI2Slot5/ai24", "PXI2Slot5/ai25", "PXI2Slot5/ai26", "PXI2Slot5/ai27", "PXI2Slot5/ai28", "PXI2Slot5/ai29", "PXI2Slot5/ai30", "PXI2Slot5/ai31", "PXI2Slot6/ai0", "PXI2Slot6/ai1", "PXI2Slot6/ai2", "PXI2Slot6/ai3", "PXI2Slot6/ai4", "PXI2Slot6/ai5", "PXI2Slot6/ai6", "PXI2Slot6/ai7", "PXI2Slot6/ai8", "PXI2Slot6/ai9", "PXI2Slot6/ai10", "PXI2Slot6/ai11", "PXI2Slot6/ai12", "PXI2Slot6/ai13", "PXI2Slot6/ai14", "PXI2Slot6/ai15", "PXI2Slot6/ai16", "PXI2Slot6/ai17", "PXI2Slot6/ai18", "PXI2Slot6/ai19", "PXI2Slot6/ai20", "PXI2Slot6/ai21", "PXI2Slot6/ai22", "PXI2Slot6/ai23", "PXI2Slot6/ai24", "PXI2Slot6/ai25", "PXI2Slot6/ai26", "PXI2Slot6/ai27", "PXI2Slot6/ai28", "PXI2Slot6/ai29", "PXI2Slot6/ai30", "PXI2Slot6/ai31", "", "PXI2Slot9/ai0", "PXI2Slot9/ai1", "PXI2Slot9/ai2", "PXI2Slot9/ai3", "PXI2Slot9/ai4", "PXI2Slot9/ai5", "PXI2Slot9/ai6", "PXI2Slot9/ai7", "PXI2Slot9/ai8", "PXI2Slot9/ai9", "PXI2Slot9/ai10", "PXI2Slot9/ai11", "PXI2Slot9/ai12", "PXI2Slot9/ai13", "PXI2Slot9/ai14", "PXI2Slot9/ai15", "PXI2Slot9/ai16", "PXI2Slot9/ai17", "PXI2Slot9/ai18", "PXI2Slot9/ai19", "PXI2Slot9/ai20", "PXI2Slot9/ai21", "PXI2Slot9/ai22", "PXI2Slot9/ai23", "PXI2Slot9/ai24", "PXI2Slot9/ai25", "PXI2Slot9/ai26", "PXI2Slot9/ai27", "PXI2Slot9/ai28", "PXI2Slot9/ai29", "PXI2Slot9/ai30", "PXI2Slot9/ai31"] ("Strings []") -> [w19] mode=indexing
        tunnel: [w18] -> w2 mode=indexing
        tunnel: "AI config" -> [w17]
        tunnel: string[] ["P_H_PT_1", "N_PT_1", "N_PT_2", "G_PT_1", "G_N_PT_1", "G_PT_Press_1", "G_PT_Press_2", "G_RTD_Bottle", "M_PT_1", "M_N_PT_1", "M_PT_Press_1", "M_PT_Press_2", "M_RTD_Bottle", "G_PT_Inj_1", "G_PT_Inj_2", "G_PT_Inj_3", "G_PT_Inj_4", "G_PT_Inj_5", "G_PT_Inj_6", "G_PT_Inj_7", "G_PT_Inj_8", "G_PT_Inj_9", "G_PT_Inj_10", "G_PT_Inj_11", "G_PT_Inj_12", "G_PT_Inj_13", "G_PT_Inj_14", "G_PT_Inj_15", "G_PT_Inj_16", "G_PT_Inj_17", "G_PT_Inj_18", "G_PT_Inj_19", "M_PT_Inj_1", "M_PT_Inj_2", "M_PT_Inj_3", "M_PT_Inj_4", "M_PT_Inj_5", "M_PT_Inj_6", "M_PT_Inj_7", "M_PT_Inj_8", "M_PT_Inj_9", "M_PT_Inj_10", "M_PT_Inj_11", "M_PT_Inj_12", "M_PT_Inj_13", "M_PT_Inj_14", "M_PT_Inj_15", "M_PT_Inj_16", "M_PT_Inj_17", "M_PT_Inj_18", "M_PT_Inj_19", "I_PT(P)_1", "I_PT(P)_2", "I_PT(P)_3", "I_PT(P)_4", "I_PT(P)_5", "I_PT(P)_6", "I_PT(P)_7", "I_PT(P)_8", "I_PT(P)_9", "I_PT(P)_10", "I_PT(P)_11", "I_PT(P)_12", "I_PT(P)_13", "I_PT(P)_14", "I_PT(P)_15", "I_PT(P)_16", "I_PT(P)_17", "I_PT(P)_18", "I_PT(P)_19", "I_PT(Red)_1", "I_PT(Red)_2", "I_PT(Red)_3", "I_PT(Red)_4", "I_PT(Red)_5", "I_PT(Red)_6", "I_PT(Red)_7", "I_PT(Red)_8", "I_PT(Red)_9", "I_PT(Red)_10", "I_PT(Red)_11", "I_PT(Red)_12", "I_PT(Red)_13", "I_PT(Red)_14", "I_PT(Red)_15", "I_PT(Red)_16", "I_PT(Red)_17", "I_PT(Red)_18", "I_PT(Red)_19"] ("appended array 2") -> [w14] mode=indexing
        i -> [w16]
        n7 = Index Array(array=w17, index=w16) -> (element=w15:T3)
        n8 = Bundle By Name(cluster=w15, "Channel_Name"=w14, "Channel_Number"=w19, "Pre_Scale_min"=0.004, "Pre_Scale_max"=0.02, "Sensor_min"=0.0, "Sensor_max"=100.0, "Units"="barg", "VI Category"="AI_C_RT") -> (w18:T3)
      }
      "AI config 2" <- w2
    }
    frame Enabled {
    }
  }
  n9 = disable-structure shown="Disabled" {
    frame Disabled {
      w23 = "%s" ("format (%s)")
      n10 = call-poly <vilib>:"Read Delimited Spreadsheet.vi"("file path (dialog if empty)"="file path (dialog if empty)", "format (%s)"=w23, "delimiter (\\t)"="," ("delimiter (\\t)")) -> ("all rows"=w26:string[][])  [unwired: 7 in, 5 out]
      "all rows" <- w26
      n11 = Replace Array Subset(array=w26, new element=string[] ["P_H_PT_1", "N_PT_1", "N_PT_2", "G_PT_1", "G_N_PT_1", "G_PT_Press_1", "G_PT_Press_2", "G_RTD_Bottle", "M_PT_1", "M_N_PT_1", "M_PT_Press_1", "M_PT_Press_2", "M_RTD_Bottle", "G_PT_Inj_1", "G_PT_Inj_2", "G_PT_Inj_3", "G_PT_Inj_4", "G_PT_Inj_5", "G_PT_Inj_6", "G_PT_Inj_7", "G_PT_Inj_8", "G_PT_Inj_9", "G_PT_Inj_10", "G_PT_Inj_11", "G_PT_Inj_12", "G_PT_Inj_13", "G_PT_Inj_14", "G_PT_Inj_15", "G_PT_Inj_16", "G_PT_Inj_17", "G_PT_Inj_18", "G_PT_Inj_19", "M_PT_Inj_1", "M_PT_Inj_2", "M_PT_Inj_3", "M_PT_Inj_4", "M_PT_Inj_5", "M_PT_Inj_6", "M_PT_Inj_7", "M_PT_Inj_8", "M_PT_Inj_9", "M_PT_Inj_10", "M_PT_Inj_11", "M_PT_Inj_12", "M_PT_Inj_13", "M_PT_Inj_14", "M_PT_Inj_15", "M_PT_Inj_16", "M_PT_Inj_17", "M_PT_Inj_18", "M_PT_Inj_19", "I_PT(P)_1", "I_PT(P)_2", "I_PT(P)_3", "I_PT(P)_4", "I_PT(P)_5", "I_PT(P)_6", "I_PT(P)_7", "I_PT(P)_8", "I_PT(P)_9", "I_PT(P)_10", "I_PT(P)_11", "I_PT(P)_12", "I_PT(P)_13", "I_PT(P)_14", "I_PT(P)_15", "I_PT(P)_16", "I_PT(P)_17", "I_PT(P)_18", "I_PT(P)_19", "I_PT(Red)_1", "I_PT(Red)_2", "I_PT(Red)_3", "I_PT(Red)_4", "I_PT(Red)_5", "I_PT(Red)_6", "I_PT(Red)_7", "I_PT(Red)_8", "I_PT(Red)_9", "I_PT(Red)_10", "I_PT(Red)_11", "I_PT(Red)_12", "I_PT(Red)_13", "I_PT(Red)_14", "I_PT(Red)_15", "I_PT(Red)_16", "I_PT(Red)_17", "I_PT(Red)_18", "I_PT(Red)_19"] ("appended array 2"), index (col)=0 ("disabled index (col)")) -> (w24:string[][])  [unwired: 1 in]
      "output array" <- w24
      n12 = disable-structure shown="Enabled" {
        disable-tunnel: w24 -> [_ _]
        disable-tunnel: w23 -> [w31 _]
        disable-tunnel: "file path (dialog if empty)" -> [w29 _]
        disable-tunnel: string[][] [["P_H_PT_1", "G_EV_Fill_HSS", "", "P_H_EV_1", "I_TC_1"], ["N_PT_1", "G_EV_Feed_HSS", "", "P_H_EV_2", "I_TC_2"], ["N_PT_2", "G_EV_Inj_E1_1_HSS", "", "P_H_EV_3", "I_TC_3"], ["G_PT_1", "", "", "G_EV_Fill", "I_TC_4"], ["G_N_PT_1", "", "", "G_EV_Feed", "I_TC_5"], ["G_PT_Press_1", "", "", "G_EPV_1", "I_TC_6"], ["G_PT_Press_2", "", "", "G_N_EPV_1", "I_TC_7"], ["G_RTD_Bottle", "", "", "M_EV_Fill", "I_TC_8"], ["M_PT_1", "", "", "M_EV_Feed", "I_TC_9"], ["M_N_PT_1", "", "", "M_EPV_1", "I_TC_10"], ["M_PT_Press_1", "", "", "M_N_EPV_1", "I_TC_11"], ["M_PT_Press_2", "", "", "G_EV_Inj_1", "I_TC_12"], ["M_RTD_Bottle", "", "", "G_EV_Inj_2", "I_TC_13"], ["G_PT_Inj_1", "", "", "G_EV_Inj_3", "I_TC_14"], ["G_PT_Inj_2", "", "", "G_EV_Inj_4", "I_TC_15"], ["G_PT_Inj_3", "", "", "G_EV_Inj_5", "I_TC_16"], ["G_PT_Inj_4", "", "", "G_EV_Inj_6", "I_TC_17"], ["G_PT_Inj_5", "", "", "G_EV_Inj_7", "I_TC_18"], ["G_PT_Inj_6", "", "", "G_EV_Inj_8", "I_TC_19"], ["G_PT_Inj_7", "", "", "G_EV_Inj_9", ""], ["G_PT_Inj_8", "", "", "R_G_EV_9", ""], ["G_PT_Inj_9", "", "", "G_EV_Inj_10", ""], ["G_PT_Inj_10", "", "", "R_G_EV_10", ""], ["G_PT_Inj_11", "", "", "G_EV_Inj_11", ""], ["G_PT_Inj_12", "", "", "R_G_EV_11", ""], ["G_PT_Inj_13", "", "", "G_EV_Inj_12", ""], ["G_PT_Inj_14", "", "", "R_G_EV_12", ""], ["G_PT_Inj_15", "", "", "G_EV_Inj_13", ""], ["G_PT_Inj_16", "", "", "R_G_EV_13", ""], ["G_PT_Inj_17", "", "", "G_EV_Inj_14", ""], ["G_PT_Inj_18", "", "", "R_G_EV_14", ""], ["G_PT_Inj_19", "", "", "G_EV_Inj_15", ""], ["M_PT_Inj_1", "", "", "R_G_EV_15", ""], ["M_PT_Inj_2", "", "", "G_EV_Inj_16", ""], ["M_PT_Inj_3", "", "", "G_EV_Inj_17", ""], ["M_PT_Inj_4", "", "", "G_EV_Inj_18", ""], ["M_PT_Inj_5", "", "", "G_EV_Inj_19", ""], ["M_PT_Inj_6", "", "", "M_EV_Inj_1", ""], ["M_PT_Inj_7", "", "", "M_EV_Inj_2", ""], ["M_PT_Inj_8", "", "", "M_EV_Inj_3", ""], ["M_PT_Inj_9", "", "", "M_EV_Inj_4", ""], ["M_PT_Inj_10", "", "", "M_EV_Inj_5", ""], ["M_PT_Inj_11", "", "", "M_EV_Inj_6", ""], ["M_PT_Inj_12", "", "", "M_EV_Inj_7", ""], ["M_PT_Inj_13", "", "", "M_EV_Inj_8", ""], ["M_PT_Inj_14", "", "", "M_EV_Inj_9", ""], ["M_PT_Inj_15", "", "", "R_M_EV_9", ""], ["M_PT_Inj_16", "", "", "M_EV_Inj_10", ""], ["M_PT_Inj_17", "", "", "R_M_EV_10", ""], ["M_PT_Inj_18", "", "", "M_EV_Inj_11", ""], ["M_PT_Inj_19", "", "", "R_M_EV_11", ""], ["I_PT(P)_1", "", "", "M_EV_Inj_12", ""], ["I_PT(P)_2", "", "", "R_M_EV_12", ""], ["I_PT(P)_3", "", "", "M_EV_Inj_13", ""], ["I_PT(P)_4", "", "", "R_M_EV_13", ""], ["I_PT(P)_5", "", "", "M_EV_Inj_14", ""], ["I_PT(P)_6", "", "", "R_M_EV_14", ""], ["I_PT(P)_7", "", "", "M_EV_Inj_15", ""], ["I_PT(P)_8", "", "", "R_M_EV_15", ""], ["I_PT(P)_9", "", "", "M_EV_Inj_16", ""], ["I_PT(P)_10", "", "", "M_EV_Inj_17", ""], ["I_PT(P)_11", "", "", "M_EV_Inj_18", ""], ["I_PT(P)_12", "", "", "M_EV_Inj_19", ""], ["I_PT(P)_13", "", "", "SP_1", ""], ["I_PT(P)_14", "", "", "SP_2", ""], ["I_PT(P)_15", "", "", "SP_3", ""], ["I_PT(P)_16", "", "", "SP_4", ""], ["I_PT(P)_17", "", "", "SP_5", ""], ["I_PT(P)_18", "", "", "SP_6", ""], ["I_PT(P)_19", "", "", "SP_7", ""], ["I_PT(Red)_1", "", "", "SP_8", ""], ["I_PT(Red)_2", "", "", "SP_9", ""], ["I_PT(Red)_3", "", "", "SP_10", ""], ["I_PT(Red)_4", "", "", "SP_11", ""], ["I_PT(Red)_5", "", "", "SP_12", ""], ["I_PT(Red)_6", "", "", "SP_13", ""], ["I_PT(Red)_7", "", "", "SP_14", ""], ["I_PT(Red)_8", "", "", "SP_15", ""], ["I_PT(Red)_9", "", "", "SP_16", ""], ["I_PT(Red)_10", "", "", "SP_17", ""], ["I_PT(Red)_11", "", "", "SP_18", ""], ["I_PT(Red)_12", "", "", "SP_19", ""], ["I_PT(Red)_13", "", "", "SP_1R", ""], ["I_PT(Red)_14", "", "", "SP_2R", ""], ["I_PT(Red)_15", "", "", "SP_3R", ""], ["I_PT(Red)_16", "", "", "SP_4R", ""], ["I_PT(Red)_17", "", "", "SP_5R", ""], ["I_PT(Red)_18", "", "", "SP_6R", ""], ["I_PT(Red)_19", "", "", "SP_7R", ""], ["", "", "", "SP_8R", ""], ["", "", "", "SP_9R", ""], ["", "", "", "SP_10R", ""], ["", "", "", "SP_11R", ""], ["", "", "", "SP_12R", ""], ["", "", "", "SP_13R", ""], ["", "", "", "SP_14R", ""], ["", "", "", "SP_15R", ""], ["", "", "", "SP_16R", ""], ["", "", "", "SP_17R", ""], ["", "", "", "SP_18R", ""], ["", "", "", "SP_19R", ""]] ("output array") -> [w28 _]
        frame Enabled {
          n13 = call-poly <vilib>:"Write Delimited Spreadsheet.vi"("file path (dialog if empty)"=w29, "format (%s)"=w31, "2D data"=w28, "delimiter (\\t)"="," ("delimiter (\\t)")) -> ()  [unwired: 10 in, 2 out]
        }
        frame Disabled {
        }
      }
    }
    frame Enabled {
    }
  }
  n14 = disable-structure shown="Enabled" {
    frame Enabled {
      n15 = for {
        N: 19 -> [_]
        tunnel: [w34] -> w33 mode=indexing
        i -> [w37]
        n16 = Increment(x=w37) -> (x+1=w36:i32)
        n17 = Number To Decimal String(number=w36) -> (decimal integer string=w35:string)  [unwired: 1 in]
        n18 = Concatenate Strings("I_PT(Red)_", w35) -> (w34:string)
      }
      "Array 4" <- w33
    }
    frame Disabled {
    }
  }
